vi "MapDryScriptActor.vi"(8 "error in (no error)":errorcluster) -> (0 "error out":errorcluster)   [LabVIEW 2017]
doc: "Use this template to build a VI to use as a subVI."
uses:
  Spectrometer Utilities/SpectrometerControllerEnum.ctl
  Spectrometer Utilities/SpectrometerCallbackdataEvent.ctl
  Spectrometer Utilities/SpectrometerData.ctl
panel:
  in  "abort":bool
  out "Measurement\nCompleted\nSuccessfully":bool
  out "Measurement\nIn\nProgress":bool
  out "Raman\nSpectrometer\nConnected":bool
  in  "Pause":bool
  in  "Stop":bool
  in  "ChooseMapPointsButton":bool caption="Choose Map \nPoints"
  in  "Start":bool
  # "Map Dry script"
  # "Number of Points Selected"
  # "[Number of Points]"
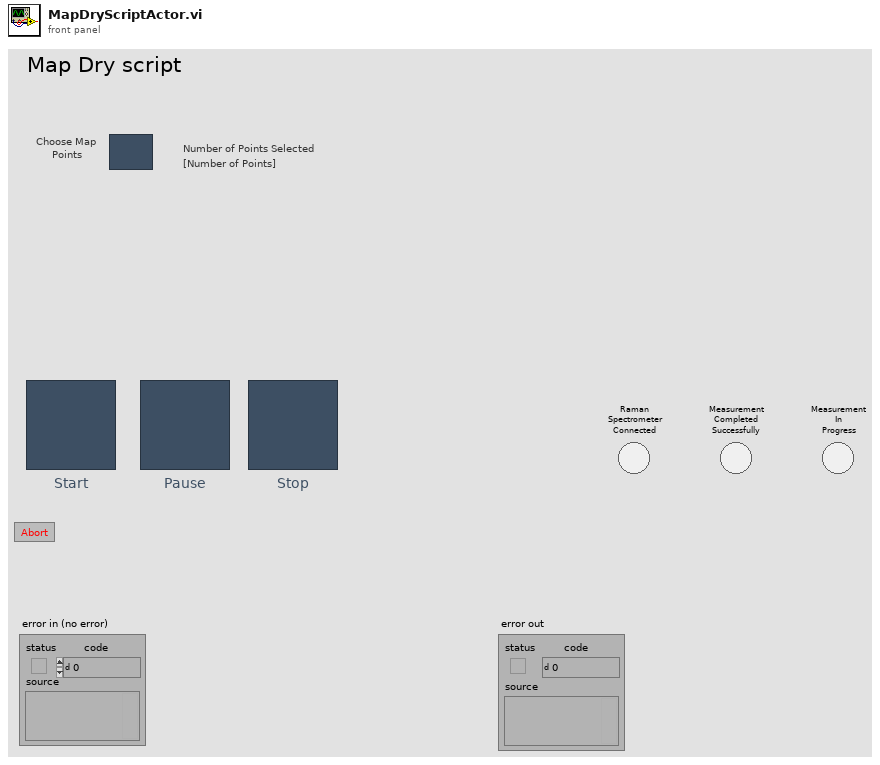
[diagram p1: front panel]
types:
  T1 = typedef "SpectrometerCallbackdataEvent.ctl" = cluster{"MeasurementEndedSuccessfully?":bool, "Spectrometer Connected?":bool, "Measurement In Progress?":bool}
  T2 = typedef "SpectrometerControllerEnum.ctl" = enum16{"Init!", "Start!", "Stop!", "Start New Measurement!", "MeasurementCompleted?", "Update Current Measurement Data", "Get Current Measurement Data!", "GetSpectrometerVIRef!", "Insert Callback Event"}
  T3 = typedef "SpectrometerData.ctl" = cluster{"Acquisition Time":dbl, "Range Begin":dbl, "Acquistion Time Unit":string, "Accumulations":i32, "Range End":dbl, "Range Unit":string, "Windows":i32, "Auto Focus":bool, "Auto Exposure":bool, "Spike Filter":string, "Delay Time":dbl, "Delay Time Unit":string, "Binning":i32, "Readout Mode":string, "DeNoise":bool, "ICS correction":bool, "Dark correction":bool, "Instrument Process":bool, "Instrument":string, "Detector":string, "Objective":string, "Grating":i32, "Grating Unit":string, "ND Filter":dbl, "ND Filter Unit":string, "Laser":dbl, "Laser Unit":string, "Slit":dbl, "Hole":dbl, "Acquired DateTime":string, "X axis":dbl[], "Y axis":dbl[]}
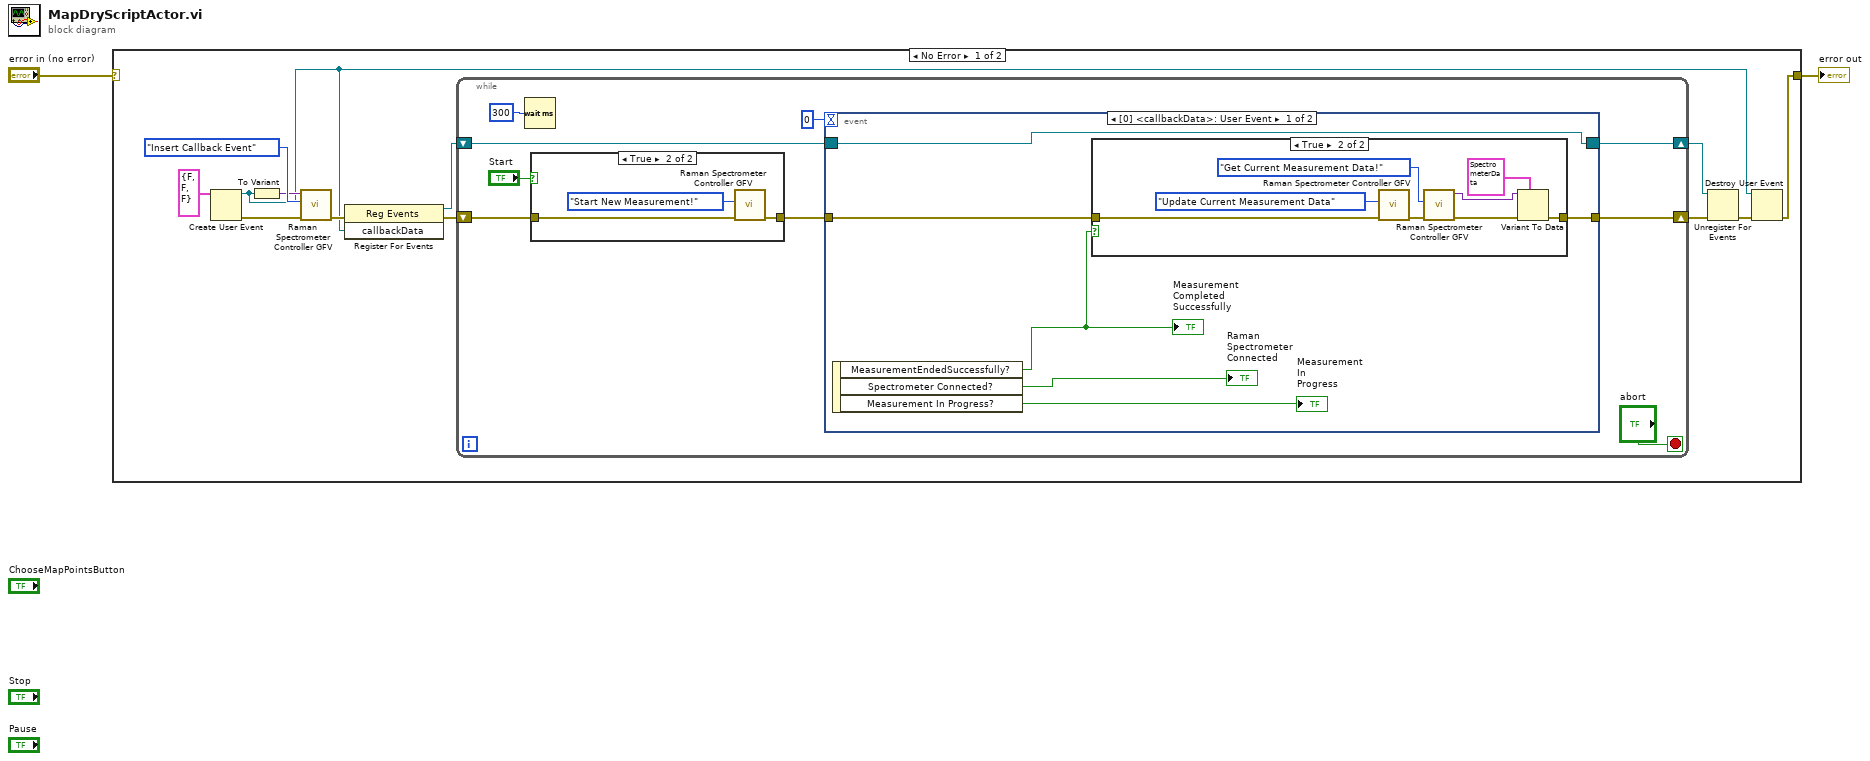
[diagram p0: block diagram]
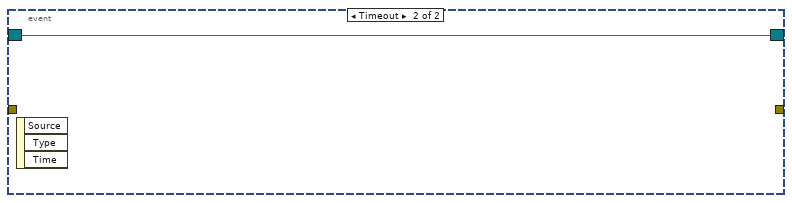
[diagram p3: hidden frame]
diagram:
  n1 = case shown="No Error" "error in (no error)" {
    selector: "error in (no error)" -> [_ w44]
    tunnel: [w3 w44] -> w1
    frame No Error {
      n2 = Create User Event(user event datatype=T1 {"MeasurementEndedSuccessfully?"=FALSE, "Spectrometer Connected?"=FALSE, "Measurement In Progress?"=FALSE} ("callbackData")) -> (user event=w5:refnum<user-event>, error out=w12:errorcluster)  [unwired: 1 in]
      n3 = To Variant(anything=w5) -> (Variant=w11:variant)
      n4 = call "Raman Spectrometer Controller GFV.vi"("Data in"=w11, "SpectrometerEnum"=SpectrometerControllerEnum."Insert Callback Event", "error in (no error)"=w12) -> ("error out"=w10:errorcluster)  [unwired: 6 in, 1 out]
      n5 = register-events(error in=w10, w5) -> (reference out=w8:refnum<event-registration>, error out=w9:errorcluster)  [unwired: 1 in]
      n6 = while {
        shift-right: [w15] -> w7
        shift-left: w9 -> [w23]
        shift-right: [w17] -> w6
        shift-left: w8 -> [w20]
        stop <- "abort" stop-if-true
        n7 = Wait (ms)(milliseconds to wait=u32 300) -> ()  [unwired: 1 out]
        n8 = case shown="True" "Start" {
          tunnel: w23 -> [w40 w43]
          tunnel: [w40 w42] -> w19
          frame False {
          }
          frame True {
            n9 = call "Raman Spectrometer Controller GFV.vi"("SpectrometerEnum"=SpectrometerControllerEnum."Start New Measurement!", "error in (no error)"=w43) -> ("error out"=w42:errorcluster)  [unwired: 7 in, 1 out]
          }
        }
        n10 = event shown="[0] <callbackData>: User Event" {
          selector: w20 -> [w27 w39]
          dyn-events: [w27 w39] -> w17
          timeout: 0 -> [_ _]
          tunnel: w19 -> [w29 _]
          tunnel: [w28 _] -> w15
          event User Event {
            n11 = event-data() -> ("MeasurementEndedSuccessfully?"=w26:bool, "Spectrometer Connected?"=→"Raman\nSpectrometer\nConnected":bool, "Measurement In Progress?"=→"Measurement\nIn\nProgress":bool)  [unwired: 1 in]
            "Measurement\nCompleted\nSuccessfully" <- w26
            n12 = case shown="True" w26 {
              tunnel: w29 -> [w30 w32]
              tunnel: [w30 w31] -> w28
              frame False {
              }
              frame True {
                n13 = call "Raman Spectrometer Controller GFV.vi"("SpectrometerEnum"=SpectrometerControllerEnum."Update Current Measurement Data", "error in (no error)"=w32) -> ("error out"=w36:errorcluster)  [unwired: 7 in, 1 out]
                n14 = call "Raman Spectrometer Controller GFV.vi"("SpectrometerEnum"=SpectrometerControllerEnum."Get Current Measurement Data!", "error in (no error)"=w36) -> ("Data Out"=w38:variant, "error out"=w37:errorcluster)  [unwired: 7 in]
                n15 = Variant To Data(error in=w37, type=T3 {"Acquisition Time"=0.0, "Range Begin"=0.0, "Acquistion Time Unit"="", "Accumulations"=0, "Range End"=0.0, "Range Unit"="", "Windows"=0, "Auto Focus"=FALSE, "Auto Exposure"=FALSE, "Spike Filter"="", "Delay Time"=0.0, "Delay Time Unit"="", "Binning"=0, "Readout Mode"="", "DeNoise"=FALSE, "ICS correction"=FALSE, "Dark correction"=FALSE, "Instrument Process"=FALSE, "Instrument"="", "Detector"="", "Objective"="", "Grating"=0, "Grating Unit"="", "ND Filter"=0.0, "ND Filter Unit"="", "Laser"=0.0, "Laser Unit"="", "Slit"=0.0, "Hole"=0.0, "Acquired DateTime"="", "X axis"=[], "Y axis"=[]} ("Spectrometer Data"), Variant=w38) -> (error out=w31:errorcluster)  [unwired: 1 out]
              }
            }
          }
          event Timeout {
            n16 = event-data() -> ()  [unwired: 1 in, 3 out]
          }
        }
      }
      n17 = Unregister For Events(event registration refnum=w6, error in=w7) -> (error out=w4:errorcluster)
      n18 = Destroy User Event(user event=w5, error in=w4) -> (error out=w3:errorcluster)
    }
    frame Error {
    }
  }
  "error out" <- w1
